vi "ReceiveEth.vi"(3 "Display":bool, 4 "queue out":refnum<queue>, 5 "Cnt in":u32, 6 "reference":refnum<vi>) -> (0 "unsigned byte array":u8[](array[numeric]), 1 "Cnt out":u32, 2 "status":bool)   [LabVIEW 2017]
panel:
  out "counter":u32
  out "error out":errorcluster
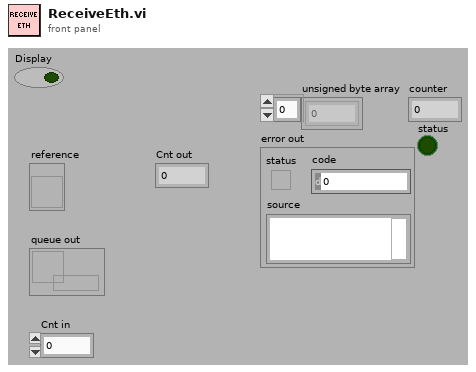
[diagram p1: front panel]
types:
  T1 = enum16{"Standard", "Buffered", "CRLF", "Immediate"}
  T2 = cluster{"ID":u32, "MSGTYPE":u8, "LEN":u8, "aDATA":u8[]}
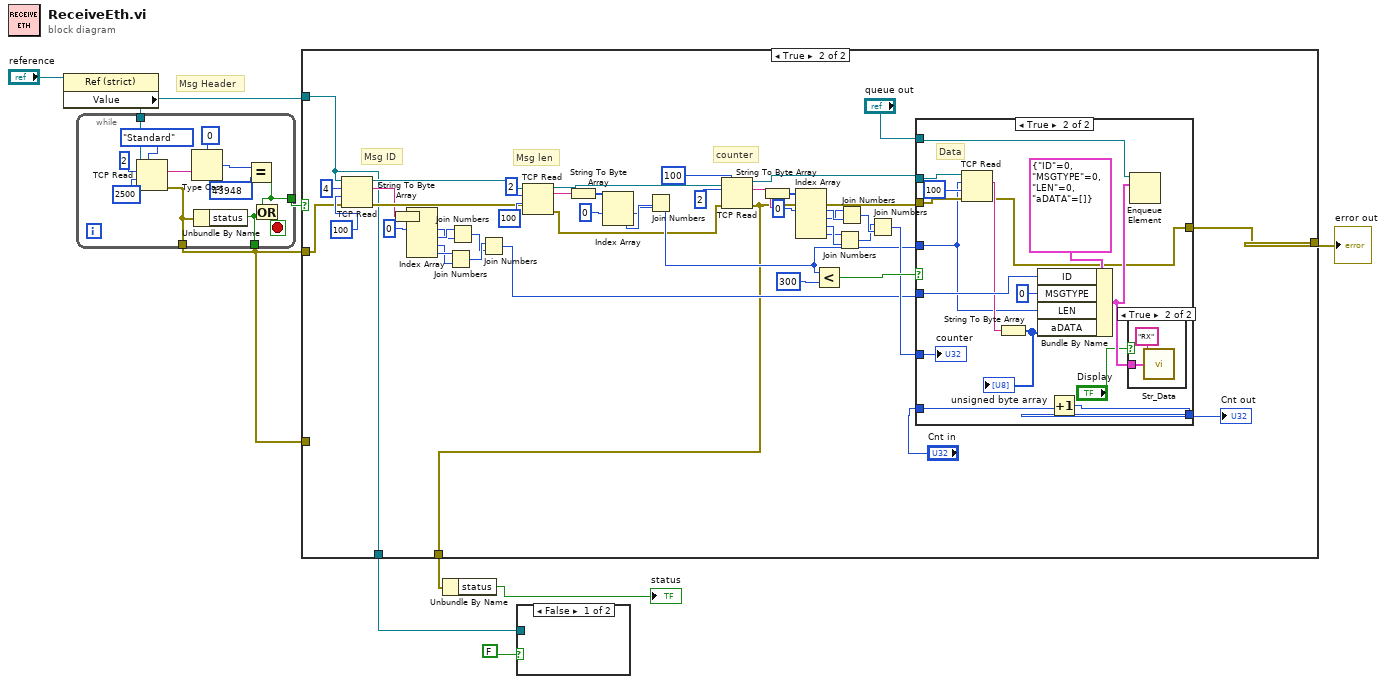
[diagram p0: block diagram]
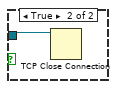
[diagram p2: hidden frame]
diagram:
  # "Msg Header"
  n1 = property class="Ref (strict)"(reference="reference") -> ("Value"=w6:refnum<k5>)  [unwired: 1 in, 2 out]
  n2 = while {
    tunnel: w6 -> [w19]
    tunnel: [w17] -> w7
    tunnel: [w11] -> w3
    tunnel: [w10] -> _
    stop <- w18 stop-if-true
    n3 = TCP Read(connection ID=w19, bytes to read=2, 7:T1."Standard" ("mode (standard)"), 9:2500) -> (data out=w15:string, error out=w11:errorcluster)  [unwired: 1 in, 1 out]
    n4 = Type Cast(type=u16 0 ("y"), x=w15) -> (*(type *) &x=w13:u16)
    n5 = Unbundle By Name(w11) -> ("status"=w10:bool)
    n6 = Equal?(x=w13, y=u16 43948) -> (x = y?=w17:bool)
    n7 = Or(x=w17, y=w10) -> (x .or. y?=w18:bool)
  }
  n8 = case shown="True" w7 {
    tunnel: w6 -> [w22 w25]
    tunnel: w3 -> [w24 w50]
    tunnel: [w24 w48] -> w8
    tunnel: [w23 w26] -> w4
    tunnel: w3 -> [w23 _]
    tunnel: [w22 w25] -> w2
    frame False {
    }
    frame True {
      # "counter"
      # "Msg ID"
      # "Msg len"
      n9 = TCP Read(connection ID=w25, bytes to read=4, error in (no error)=w50, 9:100) -> (connection ID out=w54:refnum<k5>, data out=w32:string, error out=w49:errorcluster)  [unwired: 1 in]
      n10 = String To Byte Array(string=w32) -> (unsigned byte array=w60:u8[])
      n11 = Index Array(array=w60, index #1=0 ("index")) -> (element #1=w62:u8, element #2=w63:u8, element #3=w64:u8, element #4=w65:u8)  [unwired: 3 in]
      n12 = Join Numbers(hi=w65, lo=w64) -> ((hi.lo)=w67:u16)
      n13 = Join Numbers(hi=w63, lo=w62) -> ((hi.lo)=w66:u16)
      n14 = Join Numbers(hi=w67, lo=w66) -> ((hi.lo)=w33:u32)
      n15 = TCP Read(connection ID=w54, bytes to read=2, error in (no error)=w49, 9:100) -> (connection ID out=w45:refnum<k5>, data out=w31:string, error out=w28:errorcluster)  [unwired: 1 in]
      n16 = String To Byte Array(string=w31) -> (unsigned byte array=w56:u8[])
      n17 = Index Array(array=w56, index #1=0 ("index")) -> (element #1=w57:u8, element #2=w58:u8)  [unwired: 1 in]
      n18 = Join Numbers(hi=w58, lo=w57) -> ((hi.lo)=w29:u16)
      n19 = TCP Read(connection ID=w45, bytes to read=2, error in (no error)=w28, 9:100 ("timeout ms (25000)")) -> (connection ID out=w30:refnum<k5>, data out=w44:string, error out=w26:errorcluster)  [unwired: 1 in]
      n20 = String To Byte Array(string=w44) -> (unsigned byte array=w35:u8[])
      n21 = Index Array(array=w35, index #1=0 ("index")) -> (element #1=w41:u8, element #2=w40:u8, element #3=w39:u8, element #4=w38:u8)  [unwired: 3 in]
      n22 = Less?(x=w29, y=300) -> (x < y?=w69:bool)
      n23 = Join Numbers(hi=w38, lo=w39) -> ((hi.lo)=w36:u16)
      n24 = Join Numbers(hi=w40, lo=w41) -> ((hi.lo)=w37:u16)
      n25 = Join Numbers(hi=w36, lo=w37) -> ((hi.lo)=w34:u32)
      n26 = case shown="True" w69 {
        tunnel: "queue out" -> [_ w87]
        tunnel: "Cnt in" -> [w72 w80]
        tunnel: [w72 w79] -> w70
        tunnel: w29 -> [_ w74]
        tunnel: w33 -> [_ w84]
        tunnel: w30 -> [_ w82]
        tunnel: w26 -> [w71 w77]
        tunnel: [w71 w76] -> w48
        tunnel: w34 -> [_ w75]
        frame False {
        }
        frame True {
          # "Data"
          n27 = TCP Read(connection ID=w82, bytes to read=w74, error in (no error)=w77, 9:100) -> (data out=w81:string, error out=w76:errorcluster)  [unwired: 1 in, 1 out]
          n28 = String To Byte Array(string=w81) -> (unsigned byte array=w78:u8[])
          "unsigned byte array" <- w78
          n29 = Bundle By Name(cluster=T2 {"ID"=0, "MSGTYPE"=0, "LEN"=0, "aDATA"=[]} ("Msg"), "ID"=w84, "MSGTYPE"=u8 0, "LEN"=w74, "aDATA"=w78) -> (w86:T2)
          n30 = Increment(x=w80) -> (x+1=w79:u32)
          n31 = case shown="True" "Display" {
            tunnel: w86 -> [_ w89]
            frame False {
            }
            frame True {
              n32 = call "Str_Data.vi"("Msg"=w89, "string"="RX") -> ()  [unwired: 1 in, 1 out]
            }
          }
          n33 = Enqueue Element(queue=w87, element=w86) -> ()  [unwired: 1 in, 4 out]
          "counter" <- w75
        }
      }
      "Cnt out" <- w70
    }
  }
  "error out" <- w8
  n34 = Unbundle By Name(w4) -> ("status"=→"status":bool)
  n35 = case shown="False" FALSE {
    tunnel: w2 -> [_ w91]
    frame False {
    }
    frame True {
      n36 = TCP Close Connection(connection ID=w91) -> ()  [unwired: 2 in, 2 out]
    }
  }
